vi "Reverse.vi"(8 "error in":errorcluster, 11 "Modbus instance in":refnum<class "Modbus API.lvclass">) -> (0 "error out":errorcluster, 3 "Modbus instance out":refnum<class "Modbus API.lvclass">)   [LabVIEW 2014, in "Files Library.lvlib"]
uses:
  Files Library.lvlib
  <vilib>/NI/Modbus Library/API/Modbus API.lvclass
  Global/ClockWise Global.vi
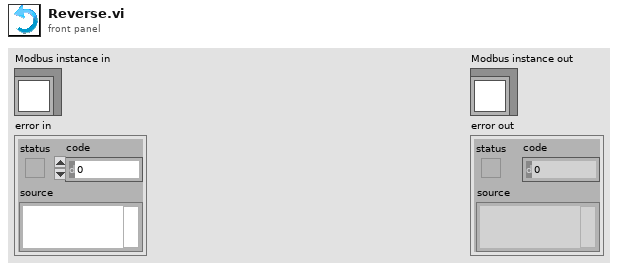
[diagram p1: front panel]
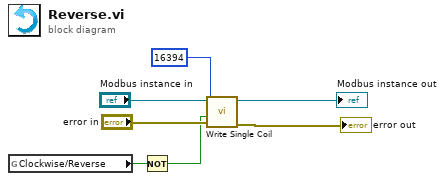
[diagram p0: block diagram]
diagram:
  n1 = global read "ClockWise Global.vi" "Clockwise/Reverse"() -> (w2:bool)
  n2 = Not(x=w2) -> (.not. x?=w1:bool)
  n3 = call-dynamic "Write Single Coil.vi"("error in"="error in", "coil to write"=w1, "address"=u16 16394, "Modbus instance in"="Modbus instance in") -> ("error out"=→"error out":errorcluster, "Modbus instance out"=→"Modbus instance out":refnum<class "Modbus API.lvclass">)  [unwired: 6 in]
